vi "ErrorLog_HasAnyErrors.vi"(8 "error in (no error)":errorcluster, 11 "reference in":refnum<class "ErrorLog.lvclass">) -> (0 "error out":errorcluster, 1 "Errors":string, 2 "Has Errors":bool, 3 "reference out":refnum<class "ErrorLog.lvclass">)   [LabVIEW 2014, in "ErrorLog.lvclass"]
uses:
  ErrorLog.lvclass
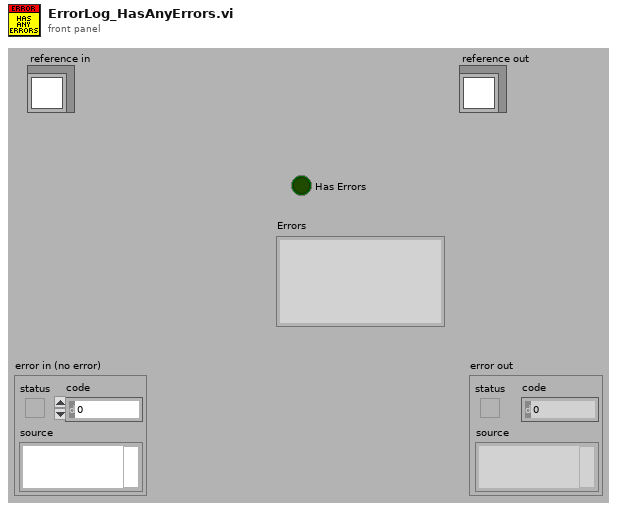
[diagram p1: front panel]
types:
  T1 = typedef "ErrorLog.lvclass/ObjectAttributes.ctl" = cluster{"ErrorFile":path, "Supress Consecutive Duplicates":bool, "Errors":string, "Quit":bool, "Errors since last call":string, "Last Recorded Error":string, "ErrorPath":path, "PossiblePaths":path[], "BaseFileName":string, "Max Log Files":i32, "ErrorFile Index":i32, "Max File Size":i64}
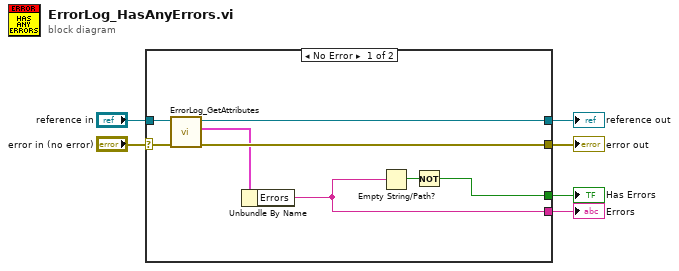
[diagram p0: block diagram]
diagram:
  n1 = case shown="No Error" "error in (no error)" {
    selector: "error in (no error)" -> [w14 w16]
    tunnel: [w12 w16] -> w5
    tunnel: [w11 w15] -> w3
    tunnel: "reference in" -> [w13 w15]
    tunnel: [w7 _] -> w2
    tunnel: [w9 _] -> w1
    frame No Error {
      n2 = call "ErrorLog_GetAttributes.vi"("error in (no error)"=w14, "reference in"=w13) -> ("error out"=w12:errorcluster, "Data"=w10:T1, "reference out"=w11:refnum<class "ErrorLog.lvclass">)  [unwired: 6 in, 1 out]
      n3 = Unbundle By Name(w10) -> ("Errors"=w9:string)
      n4 = Empty String/Path?(string/path=w9) -> (empty?=w8:bool)
      n5 = Not(x=w8) -> (.not. x?=w7:bool)
    }
    frame Error {
    }
  }
  "error out" <- w5
  "reference out" <- w3
  "Has Errors" <- w2
  "Errors" <- w1
